vi "Instantiate.vi"(1 "vi ref":refnum<vi>) -> (0 "vi ref":refnum<vi>)   [LabVIEW 2020, in "Event Messenger Priority.lvlib"]
doc: "Creates and initializes the data structure that supports the channel at run time."
uses:
  Event Messenger Priority.lvlib
  ))Channel.vi
  ChannelOp.ctl
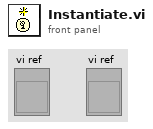
[diagram p1: front panel]
types:
  T1 = typedef "Event Messenger Priority.lvlib/ChannelOp.ctl" = enum16{"init", "write", "register", "replicate", "probe"}
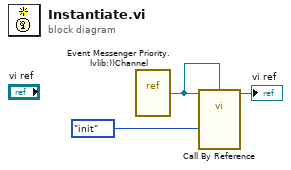
[diagram p0: block diagram]
diagram:
  n1 = vi-ref "Event Messenger Priority.lvlib:))Channel.vi"() -> (w2:refnum<vi>)
  n2 = call-by-ref "?"(reference=w2, "This VI"=w2, "channelOp"=ChannelOp."init") -> (reference out=→"vi ref":refnum<vi>)  [unwired: 10 in, 6 out]
